vi "Reaffirm_ADAM_Outputs.vi"(3 "Channel Description":T1[](array[typedef]) {"Duty" format="%.0b"; "D" format="%#_5g"; "C" format="%#_5g"; "B" format="%#_5g"; "A" format="%#_5g"}, 4 "Active Ch Indicies":i32[](array[numeric]), 5 "Current Channel Values":dbl[](array[numeric]) format="%.2f") -> (1 "Scan Comments":string[](array[string]))   [LabVIEW 2011]
uses:
  ADAM Client/Sub VIs/ADAM Controls/Ch_description_ADAM.ctl
  ADAM Client/Sub VIs/ADAM Controls/Module_type_ADAM.ctl
  ADAM Client/Sub VIs/ADAM Controls/Function_ADAM.ctl
  ADAM Client/Sub VIs/ADAM Controls/Channel_State.ctl
  ADAM Client/Sub VIs/ADAM Controls/Calib_type_ADAM.ctl
  ADAM Client/Sub VIs/ADAM Controls/Address.ctl
  ADAM_Global.vi
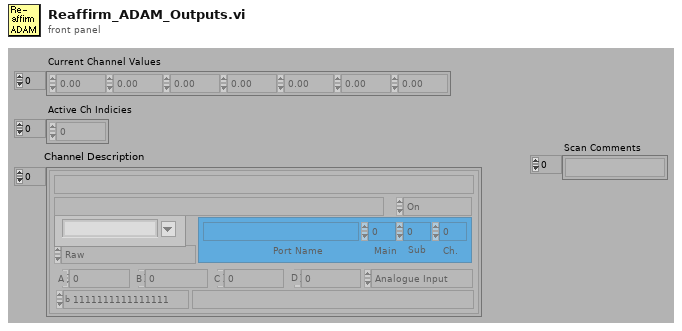
[diagram p1: front panel]
types:
  T1 = typedef "Ch_description_ADAM.ctl" = cluster{"Ch Name":string, "Type":T2, "Function":T3, "Ch State":T4, "Calibration type":T5, "A":dbl, "B":dbl, "C":dbl, "D":dbl, "Comments":string, "Address":T6, "String":string, "Duty":u16}
  T2 = typedef "Module_type_ADAM.ctl" = string
  T3 = typedef "Function_ADAM.ctl" = enum16{"Analogue Input", "Digital Input", "Event counter", "Event rate", "Analogue Output", "Digital Output", "Relay Output"}
  T4 = typedef "Channel_State.ctl" = enum16{"On", "Off", "Always On", "Always Off"}
  T5 = typedef "Calib_type_ADAM.ctl" = enum16{"Raw", "Bx + A", "Cx^2 + Bx + A", "Dx^3 + Cx^2 + Bx + A", "In Band", "Hi-Tec Q", "Hi-Tec M_dot", "Text"}
  T6 = typedef "Address.ctl" = cluster{"Main":i32, "Ch.":i32, "Sub":i32, "Port Name":string}
  T7 = typedef "Server_Control.ctl" = cluster{"Channel Name to control":string, "Channel sharing":enum16{"Channel Unshared", "Channel Shared by Rig", "Channel Shared by Group"}, "Default Value":dbl, "Client Array":string[], "Time Stamp":timestamp, "Do Not Reset":bool}
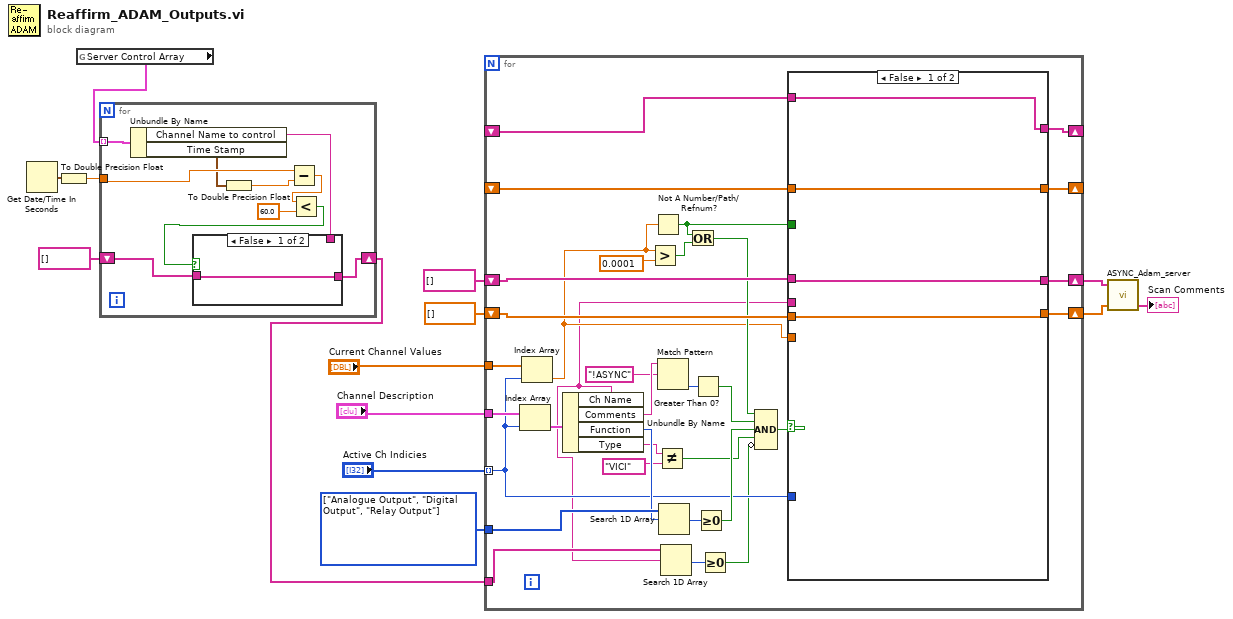
[diagram p0: block diagram]
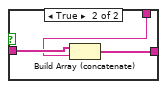
[diagram p2: hidden frame]
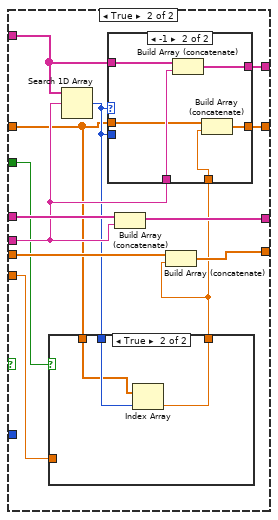
[diagram p3: hidden frame]
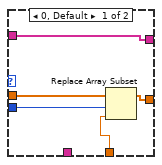
[diagram p4: hidden frame]
diagram:
  w12 = T3[] [enum."Analogue Output", enum."Digital Output", enum."Relay Output"] items=["Analogue Input", "Digital Input", "Event counter", "Event rate", "Analogue Output", "Digital Output", "Relay Output"]
  n1 = Get Date/Time In Seconds() -> (seconds since 1Jan1904=w4:timestamp)
  n2 = To Double Precision Float(number=w4) -> (double precision float=w3:dbl)
  n3 = global read "ADAM_Global.vi" "Server Control Array"() -> (w5:T7[])
  n4 = for {
    tunnel: w5 -> [w24] mode=indexing
    tunnel: w3 -> [w23]
    shift-right: [w16] -> w1
    shift-left: string[] [] -> [w17]
    n5 = Unbundle By Name(w24) -> ("Channel Name to control"=w15:string, "Time Stamp"=w22:timestamp)
    n6 = To Double Precision Float(number=w22) -> (double precision float=w21:dbl)
    n7 = Subtract(x=w23, y=w21) -> (x-y=w20:dbl)
    n8 = Less?(x=w20, y=60.0) -> (x < y?=w18:bool)
    n9 = case shown="False" w18 {
      tunnel: w17 -> [w25 w28]
      tunnel: [w25 w27] -> w16
      tunnel: w15 -> [_ w26]
      frame False {
      }
      frame True {
        n10 = Build Array (concatenate)(w28, w26) -> (w27:string[])
      }
    }
  }
  n11 = for {
    tunnel: "Channel Description" -> [w51]
    tunnel: "Active Ch Indicies" -> [w45] mode=indexing
    tunnel: w12 -> [w60]
    shift-right: [w49] -> w7
    shift-left: dbl[] [] -> [w50]
    shift-right: [w48] -> w8
    shift-left: string[] [] -> [w47]
    tunnel: "Current Channel Values" -> [w46]
    shift-right: [w39] -> _
    shift-left: _ -> [w40]
    shift-right: [w37] -> _
    shift-left: _ -> [w38]
    tunnel: w1 -> [w32]
    n12 = Index Array(array=w51, index=w45) -> (element=w61:T1)
    n13 = Index Array(array=w46, index=w45) -> (element=w35:dbl)
    n14 = Unbundle By Name(w61) -> ("Ch Name"=w31:string, "Comments"=w58:string, "Function"=w59:T3, "Type"=w43:T2)
    n15 = Greater?(x=w35, y=0.0001) -> (0:w34:bool)
    n16 = Not A Number/Path/Refnum?(number/path/refnum=w35) -> (NaN/Path/Refnum?=w33:bool)
    n17 = Not Equal?(x=w43, y=T2 "VICI" ("Type")) -> (x != y?=w41:bool)
    n18 = Match Pattern(string=w58, regular expression="!ASYNC") -> (offset past match=w56:i32)  [unwired: 4 out]
    n19 = Search 1D Array(1D array=w60, element=w59) -> (index of element=w55:i32)  [unwired: 1 out]
    n20 = Search 1D Array(1D array=w32, element=w31) -> (index of element=w30:i32)  [unwired: 1 out]
    n21 = Or(x=w33, y=w34) -> (x .or. y?=w36:bool)
    n22 = Greater Than 0?(x=w56) -> (x > 0?=w53:bool)
    n23 = Greater Or Equal To 0?(x=w55) -> (x >= 0?=w54:bool)
    n24 = Greater Or Equal To 0?(x=w30) -> (x >= 0?=w29:bool)
    n25 = Compound Arithmetic op=AND(w36, w53, w54, w41, invert w29) -> (w52:bool)
    n26 = case shown="False" w52 {
      tunnel: w45 -> [_ _]
      tunnel: w50 -> [w64 w78]
      tunnel: [w64 w77] -> w49
      tunnel: w31 -> [_ w73]
      tunnel: [w65 w76] -> w48
      tunnel: w47 -> [w65 w75]
      tunnel: w35 -> [_ w70]
      tunnel: w40 -> [w63 w74]
      tunnel: [w63 w72] -> w39
      tunnel: w38 -> [w62 w68]
      tunnel: [w62 w71] -> w37
      tunnel: w33 -> [_ w66]
      frame False {
      }
      frame True {
        n27 = Search 1D Array(1D array=w74, element=w73) -> (index of element=w69:i32)  [unwired: 1 out]
        n28 = case shown="True" w66 {
          tunnel: [w90 w91] -> w67
          tunnel: w70 -> [w90 _]
          tunnel: w69 -> [_ w93]
          tunnel: w68 -> [_ w92]
          frame False {
          }
          frame True {
            n29 = Index Array(array=w92, index=w93) -> (element=w91:dbl)
          }
        }
        n30 = case shown="-1" w69 {
          tunnel: w74 -> [w83 w89]
          tunnel: w73 -> [_ w88]
          tunnel: [w83 w87] -> w72
          tunnel: w69 -> [w82 _]
          tunnel: w68 -> [w81 w86]
          tunnel: [w80 w84] -> w71
          tunnel: w67 -> [w79 w85]
          frame 0, Default {
            n31 = Replace Array Subset(array=w81, new element=w79, index=w82) -> (w80:dbl[])
          }
          frame -1 {
            n32 = Build Array (concatenate)(w89, w88) -> (w87:string[])
            n33 = Build Array (concatenate)(w86, w85) -> (w84:dbl[])
          }
        }
        n34 = Build Array (concatenate)(w75, w73) -> (w76:string[])
        n35 = Build Array (concatenate)(w78, w67) -> (w77:dbl[])
      }
    }
  }
  n36 = call "ASYNC_Adam_server.vi"("Values"=w7, "Channel Names"=w8) -> ("Scan Comments"=→"Scan Comments":string[])  [unwired: 1 in, 2 out]
